vi "Read.vi"(8 "error in (no error)":errorcluster, 11 "queue":refnum<queue>) -> (0 "error out":errorcluster, 1 "payload":string, 2 "state":string, 3 "queue out":refnum<queue>)   [LabVIEW 2019, in "Simple Queue Message.lvlib"]
uses:
  Simple Queue Message.lvlib
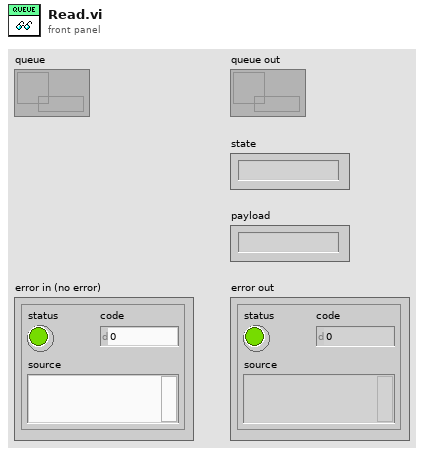
[diagram p1: front panel]
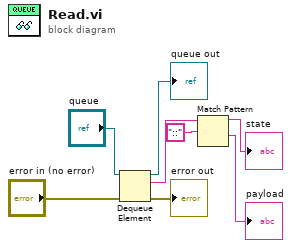
[diagram p0: block diagram]
diagram:
  n1 = Dequeue Element(queue="queue", error in (no error)="error in (no error)") -> (queue out=→"queue out":refnum<queue>, element=w4:string, error out=→"error out":errorcluster)  [unwired: 1 in, 1 out]
  n2 = Match Pattern(string=w4, regular expression="::") -> (before substring=→"state":string, after substring=→"payload":string)  [unwired: 1 in, 2 out]
